vi "Read Value (variant).vi"(8 "error in (no error)":errorcluster, 11 "U8 D Element in":refnum<class "U8 D Element.lvclass">) -> (0 "error out":errorcluster, 2 "Variant":variant, 3 "U8 D Element out":refnum<class "U8 D Element.lvclass">)   [LabVIEW 2018, in "D Datagrid Library.lvlib" / "U8 D Element.lvclass"]
uses:
  U8 D Element.lvclass
  U8 D Element.lvclass/U8 D Element.ctl
  Read Value.vi
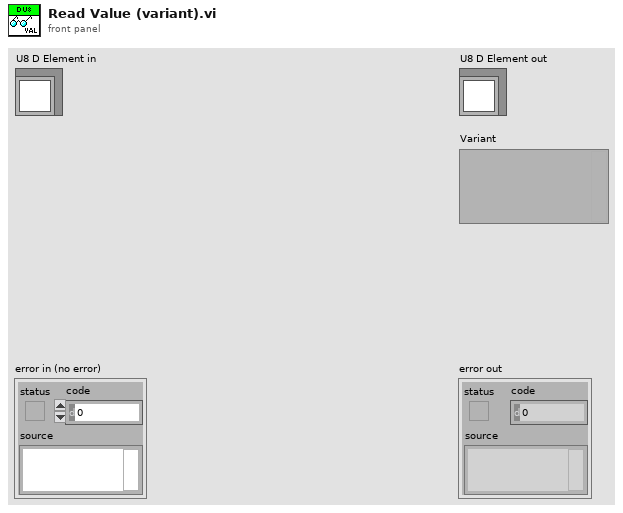
[diagram p1: front panel]
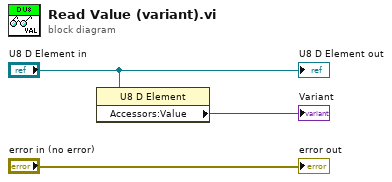
[diagram p0: block diagram]
diagram:
  n1 = property class="U8 D Element"(reference="U8 D Element in") -> ("Accessors:Value"=→"Variant":u8)  [unwired: 1 in, 2 out]
  "error out" <- "error in (no error)"
  "U8 D Element out" <- "U8 D Element in"
